vi "File_setup.vi"(4 "Measurement is top level?":bool, 5 "Results file":path, 6 "Raw data file":path, 7 "setup":T1, 8 "File":T3) -> (0 "Results file output":path, 1 "Raw data file output":path, 2 "Raw data option":enum16{"Save raw data", "Raw data not saved"}(ring), 3 "File output":T2(ring))   [LabVIEW 2020]
uses:
  Controls/Save_Data.ctl
  Controls/Setup.ctl
  Controls/Post_Process.ctl
  Globals/Meas_global.vi
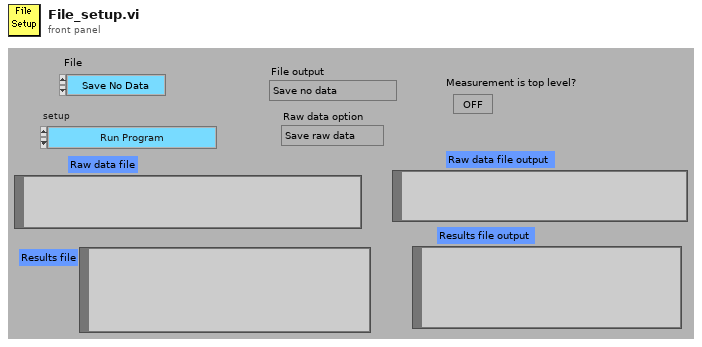
[diagram p1: front panel]
types:
  T1 = typedef "Setup.ctl" = enum16{"Run Program", "Show Setup", "Save Current Setup", "Setup Front Panel"}
  T2 = enum16{"Save no data", "Save data in new files", "Save data in existing files"}
  T3 = typedef "Save_Data.ctl" = enum16{"Save No Data", "Save Data"}
  T4 = typedef "Post_Process.ctl" = enum16{"Take New Data", "Post Process Raw Data File"}
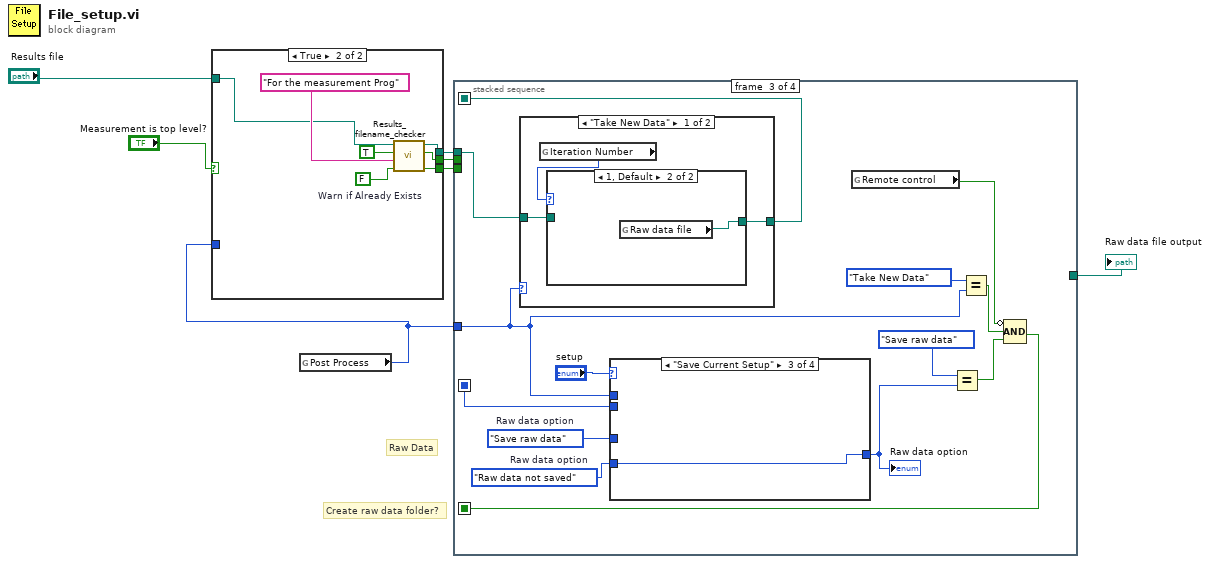
[diagram p0: block diagram]
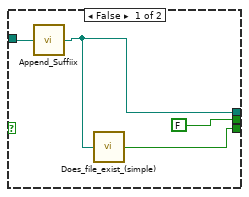
[diagram p2: hidden frame]
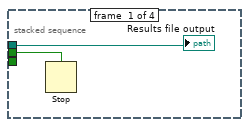
[diagram p3: hidden frame]
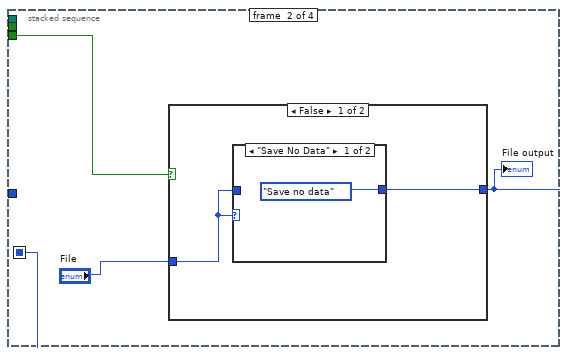
[diagram p4: hidden frame]
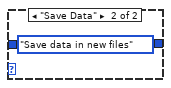
[diagram p5: hidden frame]
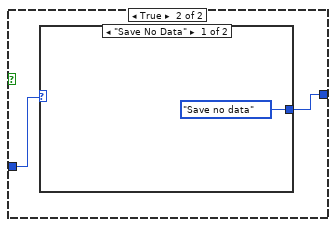
[diagram p6: hidden frame]
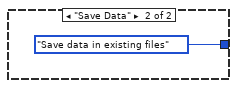
[diagram p7: hidden frame]
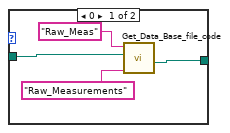
[diagram p8: hidden frame]
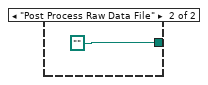
[diagram p9: hidden frame]
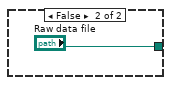
[diagram p17: hidden frame]
diagram:
  # "Create raw data folder?"
  # "Raw Data"
  n1 = global read "Meas_global.vi" "Post Process"() -> (w3:T4)
  n2 = case shown="True" "Measurement is top level?" {
    tunnel: [w9 w18] -> w7
    tunnel: [w11 w17] -> w6
    tunnel: [FALSE ("cancelled") w16] -> w4
    tunnel: w3 -> [_ _]
    tunnel: "Results file" -> [w8 w12]
    frame False {
      n3 = call "Append_Suffiix.vi"("Results file"=w8) -> ("appended path"=w9:path)
      n4 = call "Does_file_exist_(simple).vi"("Pathname"=w9) -> ("exists?"=w11:bool)
    }
    frame True {
      w13 = FALSE  # Warn if Already Exists
      n5 = call "Results_filename_checker.vi"("Warn if Already Exists"=w13, "Comment"="For the measurement Prog", "Show Error handler"=TRUE, "Results file"=w12) -> ("exists?"=w17:bool, "cancelled"=w16:bool, "Results file output"=w18:path)  [unwired: 1 in, 1 out]
    }
  }
  n6 = stacked-sequence {
    seq-local: [_ w22 _ _] -> [_ _ w45 _]
    seq-local: [_ _ w36 _] -> [_ _ _ w73]
    seq-local: [_ _ w32 _] -> [_ _ _ w71]
    tunnel: w3 -> [_ _ w33 _]
    tunnel: w7 -> [w20 _ w35 w74]
    tunnel: w6 -> [_ w21 _ _]
    tunnel: [_ _ _ w72] -> w5
    tunnel: w4 -> [w19 _ _ _]
    frame #0 {
      n7 = Stop(stop? (T)=w19) -> ()
      "Results file output" <- w20
    }
    frame #1 {
      n8 = case shown="False" w21 {
        tunnel: "File" -> [w24 w29]
        tunnel: [w25 w28] -> w22
        frame False {
          n9 = case shown="\"Save No Data\"" w24 {
            tunnel: [T2."Save no data" ("File output") T2."Save data in new files" ("File output")] -> w25
            tunnel: w24 -> [_ _]
            frame "Save No Data" {
            }
            frame "Save Data" {
            }
          }
        }
        frame True {
          n10 = case shown="\"Save No Data\"" w29 {
            tunnel: [T2."Save no data" ("File output") T2."Save data in existing files" ("File output")] -> w28
            frame "Save No Data" {
            }
            frame "Save Data" {
            }
          }
        }
      }
      "File output" <- w22
    }
    frame #2 {
      w43 = enum16{"Save raw data", "Raw data not saved"}."Raw data not saved"  # Raw data option
      w44 = enum16{"Save raw data", "Raw data not saved"}."Save raw data"  # Raw data option
      n11 = case shown="\"Take New Data\"" w33 {
        tunnel: w35 -> [w48 _]
        tunnel: [w47 path ""] -> w32
        frame "Take New Data" {
          n12 = global read "Meas_global.vi" "Iteration Number"() -> (w46:i32)
          n13 = case shown="1, Default" w46 {
            tunnel: w48 -> [w52 _]
            tunnel: [w51 w53] -> w47
            frame 0 {
              n14 = call "Get_Data_Base_file_code.vi"("Data Type"="Raw_Measurements", "Results Filename"=w52, "Short_Name"="Raw_Meas") -> ("Raw Data File Name"=w51:path)  [unwired: 1 in, 3 out]
            }
            frame 1, Default {
              n15 = global read "Meas_global.vi" "Raw data file"() -> (w53:path)
            }
          }
        }
        frame "Post Process Raw Data File" {
        }
      }
      n16 = case shown="\"Save Current Setup\"" "setup" {
        tunnel: [w59 w68 w69 w70] -> w41
        tunnel: w43 -> [w58 w68 w69 w70]
        tunnel: w44 -> [w57 _ _ _]
        tunnel: w33 -> [w56 _ _ _]
        tunnel: w45 -> [w55 _ _ _]
        frame "Run Program" {
          n17 = case shown="\"Take New Data\"" w56 {
            tunnel: w55 -> [w63 _]
            tunnel: [w62 w67] -> w59
            tunnel: w57 -> [w61 _]
            tunnel: w58 -> [w60 w67]
            frame "Take New Data" {
              n18 = case shown="\"Save no data\"" w63 {
                tunnel: [w64 w65 w66] -> w62
                tunnel: w60 -> [w64 _ _]
                tunnel: w61 -> [_ w65 w66]
                frame "Save no data" {
                }
                frame "Save data in new files" {
                }
                frame "Save data in existing files" {
                }
              }
            }
            frame "Post Process Raw Data File" {
            }
          }
        }
        frame "Show Setup" {
        }
        frame "Save Current Setup" {
        }
        frame "Setup Front Panel" {
        }
      }
      "Raw data option" <- w41
      n19 = global read "Meas_global.vi" "Remote control"() -> (w34:bool)
      n20 = Equal?(x=enum16{"Save raw data", "Raw data not saved"}."Save raw data" ("Raw data option"), y=w41) -> (x = y?=w38:bool)
      n21 = Equal?(x=Post_Process."Take New Data" ("Post Process"), y=w33) -> (x = y?=w37:bool)
      n22 = Compound Arithmetic op=AND(invert w34, w37, w38) -> (w36:bool)
    }
    frame #3 {
      n23 = case shown="True" w73 {
        tunnel: [w75 "Raw data file"] -> w72
        tunnel: w74 -> [_ _]
        tunnel: w71 -> [w75 _]
        frame True {
        }
        frame False {
        }
      }
    }
  }
  "Raw data file output" <- w5
